vi "SUB_Questionaire.vi"() -> (0 "color":T1(ring))   [LabVIEW 2011]
doc: "This is an example of how to use the radio buttons control with the Value Changed event."
panel:
  in  "What Color did you see on Display ?":T1(radio)=enum."None"
  # "請用鼠標點選剛待測物顯示的顏色. 如果LCD NG 請選Fail"
  # "需檢測壞點.如LCD 是NG點選Fail選項"
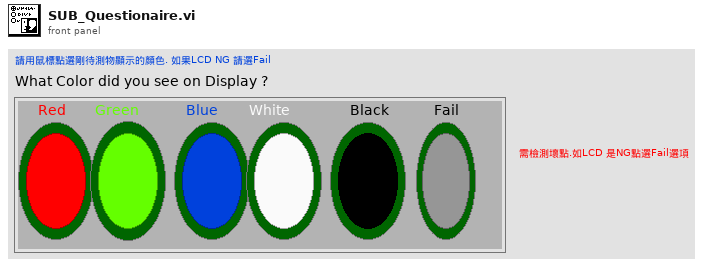
[diagram p1: front panel]
types:
  T1 = enum32{"No Selection", "None", "Red", "Green", "Blue", "White", "Black", "Fail"}
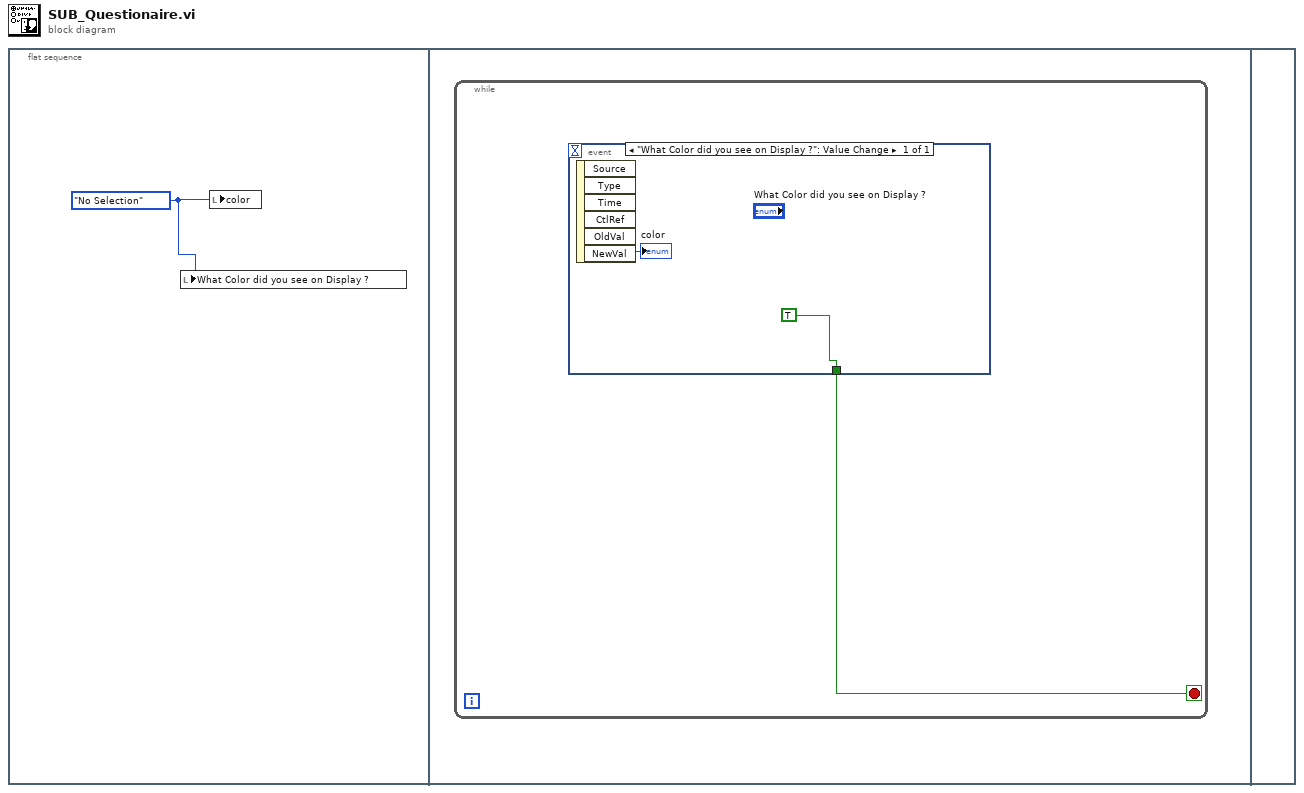
[diagram p0: block diagram]
diagram:
  n1 = flat-sequence {
    frame #0 {
      w1 = T1."No Selection" ("color")
      n2 = local write "What Color did you see on Display ?"(w1) -> ()
      n3 = local write "color"(w1) -> ()
    }
    frame #1 {
      n4 = while {
        stop <- w2 stop-if-true
        n5 = event shown="[0] \"What Color did you see on Display ?\": Value Change" {
          selector: _ -> [_]
          dyn-events: _ -> [_]
          timeout: _ -> [_]
          tunnel: [TRUE] -> w2
          event "What Color did you see on Display ?": Value Change {
            n6 = event-data() -> ("NewVal"=→"color":T1)  [unwired: 1 in, 5 out]
          }
        }
      }
    }
    frame #2 {
    }
  }
